vi "GUI Controller Performace Window.vi"() -> ()   [LabVIEW 2011, in "User Interface Window VIs.lvlib"]
uses:
  User Interface Window VIs.lvlib
  Types Definitions/Type Diagnostics Sample.ctl
  Types Definitions/Type Diagnostics Data.ctl
  Types Definitions/Type CPU Loads Array.ctl
  Types Definitions/Type CPU Loads.ctl
  Types Definitions/Type Configuration Data (GUI to Controller).ctl
  Types Definitions/Type FOFB Parameters.ctl
  Types Definitions/Type Network Configuration.ctl
  Types Definitions/Type FA Configuration.ctl
  Types Definitions/Type Response Matrix Measurement Configuration.ctl
  Types Definitions/Type Correction Algorithm Configuration.ctl
  Types Definitions/Type Acquisition Network Configuration.ctl
  Types Definitions/Type Actuation Network Configuration.ctl
  <vilib>/express/express shared/transition.llb/Dynamic To Waveform Array.vi
  <vilib>/express/express signal manip/GetorSetDDTAttributes/Set DDT Attributes/SetT0.vi
  <vilib>/express/express shared/transition.llb/Waveform Array To Dynamic.vi
  <vilib>/express/express signal manip/GetorSetDDTAttributes/Set DDT Attributes/Set DDT Properties.xnode
  Type Definitions.lvlib
panel:
  in  "Tab Control":T1(tab)
  out "Memory":dynamicdata(graph)=[{"t0"=timestamp(3442295670.8960543 s since 1904-01-01), "dt"=1.0, "Y"=[979.33984375], "attributes"=variant("NI_ExpTimeStamp"=variant(timestamp timestamp(3442295670.8960543 s since 1904-01-01)))}]
  out "Missed Iterations":dynamicdata(graph)=[{"t0"=timestamp(3442295670.8960543 s since 1904-01-01), "dt"=1.0, "Y"=[335.0], "attributes"=variant("NI_ExpTimeStamp"=variant(timestamp timestamp(3442295670.8960543 s since 1904-01-01)))}]
  out "CPU":dynamicdata(graph)=[{"t0"=timestamp(3442295670.8960543 s since 1904-01-01), "dt"=1.0, "Y"=[73.75901717969012], "attributes"=variant("NI_ExpTimeStamp"=variant(timestamp timestamp(3442295670.8960543 s since 1904-01-01)))}, {"t0"=timestamp(3442295670.8960543 s since 1904-01-01), "dt"=1.0, "Y"=[51.210817049644916], "attributes"=variant("NI_ExpTimeStamp"=variant(timestamp timestamp(3442295670.8960543 s since 1904-01-01)))}, {"t0"=timestamp(3442295670.8960543 s since 1904-01-01), "dt"=1.0, "Y"=[21.886355480263205], "attributes"=variant("NI_ExpTimeStamp"=variant(timestamp timestamp(3442295670.8960543 s since 1904-01-01)))}, {"t0"=timestamp(3442295670.8960543 s since 1904-01-01), "dt"=1.0, "Y"=[0.0], "attributes"=variant("NI_ExpTimeStamp"=variant(timestamp timestamp(3442295670.8960543 s since 1904-01-01)))}, {"t0"=timestamp(3442295670.8960543 s since 1904-01-01), "dt"=1.0, "Y"=[31.473643386938022], "attributes"=variant("NI_ExpTimeStamp"=variant(timestamp timestamp(3442295670.8960543 s since 1904-01-01)))}, {"t0"=timestamp(3442295670.8960543 s since 1904-01-01), "dt"=1.0, "Y"=[0.5343387174557266], "attributes"=variant("NI_ExpTimeStamp"=variant(timestamp timestamp(3442295670.8960543 s since 1904-01-01)))}, {"t0"=timestamp(3442295670.8960543 s since 1904-01-01), "dt"=1.0, "Y"=[30.632623496579622], "attributes"=variant("NI_ExpTimeStamp"=variant(timestamp timestamp(3442295670.8960543 s since 1904-01-01)))}, {"t0"=timestamp(3442295670.8960543 s since 1904-01-01), "dt"=1.0, "Y"=[0.0], "attributes"=variant("NI_ExpTimeStamp"=variant(timestamp timestamp(3442295670.8960543 s since 1904-01-01)))}]
  out "Execution Time":dynamicdata(graph)=[{"t0"=timestamp(3442295670.8960543 s since 1904-01-01), "dt"=1.0, "Y"=[0.0], "attributes"=variant("NI_ExpTimeStamp"=variant(timestamp timestamp(3442295670.8960543 s since 1904-01-01)))}]
  in  "Send RT Execution Trace Request":bool
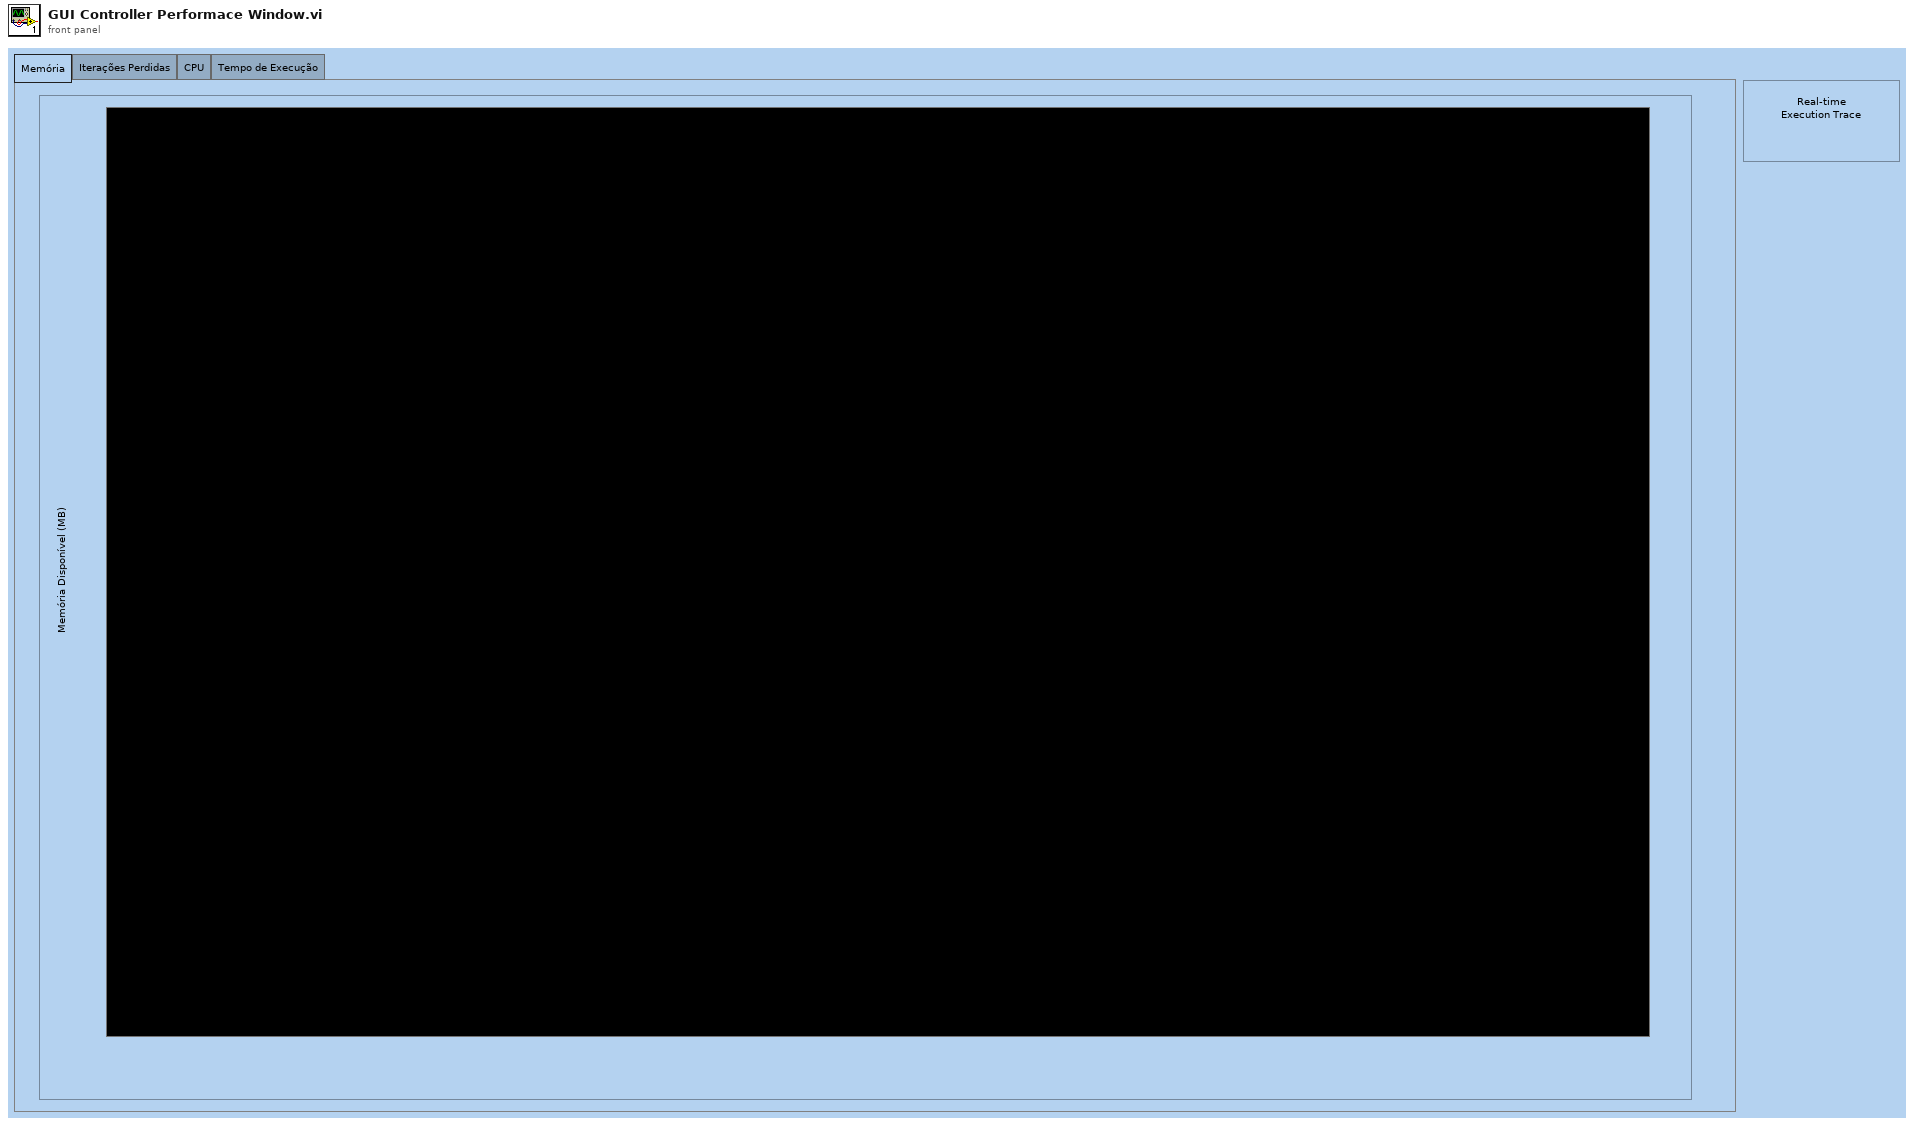
[diagram p1: front panel]
types:
  T1 = enum32{"Memória", "Iterações Perdidas", "CPU", "Tempo de Execução"}
  T2 = typedef "Type Definitions.lvlib/Type Configuration Data (GUI to Controller).ctl" = cluster{"Update Controller Soft Configuration":bool[], "Trigger RT Execution Trace":string[], "Reference Orbit":dbl[], "Request Response Matrix Folder List":bool[], "Request FOFB Parameters":bool[], "FOFB Parameters":T3[]}
  T3 = typedef "Type Definitions.lvlib/Type FOFB Parameters.ctl" = cluster{"Network":T4, "Fast Acquisition":T5, "Response Matrix Measurement":T6, "Correction Algorithm":T7, "Acquisition Network":T8, "Actuation Network":T9}
  T4 = typedef "Type Definitions.lvlib/Type Network Configuration.ctl" = cluster{"FOFB Controller IP":string, "LNLS Control Network IP":string, "LNLS Control Network Power Supplies TCP Port":u16, "LNLS Control Network FOFB Configuration TCP Port":u16, "Data Server TCP Port":u16, "Monitoring Data TCP Port":u16, "Configuration GUI TCP Port":u16, "TCP Listening Timeout":i32}
  T5 = typedef "Type Definitions.lvlib/Type FA Configuration.ctl" = cluster{"Acquisition Period":u32, "Data Buffer Size":u32, "Monitoring Period":u32}
  T6 = typedef "Type Definitions.lvlib/Type Response Matrix Measurement Configuration.ctl" = cluster{"Step Amplitude":dbl, "Time Between Steps":u32, "Step Duration":u32, "Number of Averages":u32}
  T7 = typedef "Type Definitions.lvlib/Type Correction Algorithm Configuration.ctl" = cluster{"Correction Period":u32, "Reference Orbit Path":path, "Response Matrix Path":path, "Correction Matrix Path":path, "Horizontal Correction Factor":dbl, "Vertical Correction Factor":dbl, "Beam Current FOFB Threshold":dbl, "Decouple H-V":bool, "Use Additional BPM LPF":bool, "BPM LPF Cutoff":dbl}
  T8 = typedef "Type Definitions.lvlib/Type Acquisition Network Configuration.ctl" = cluster{"Chassis Name":string, "Variables":cluster{"Variable Name":string, "Matrix Order":u32, "Location":dbl, "Plane":enum8{"H", "V"}, "On Correction":bool}[]}[]
  T9 = typedef "Type Definitions.lvlib/Type Actuation Network Configuration.ctl" = cluster{"Chassis Name":string, "Variables":cluster{"Variable Name":string, "Matrix Order":u32, "RMM Step Factor":dbl, "Plane":enum8{"H", "V"}, "On Correction":bool, "Kc":dbl, "Ti":dbl, "Td":dbl}[]}[]
  T10 = typedef "Type Definitions.lvlib/Type Diagnostics Sample.ctl" = cluster{"Timestamp":timestamp, "Diagnostics Data":T11}
  T11 = typedef "Type Definitions.lvlib/Type Diagnostics Data.ctl" = cluster{"Time-Critical Loop Missed Iterations":u32, "Time-Critical Loop Execution Time (usec)":u32, "FA Buffer Usage":u32, "Available Memory (bytes)":u32, "CPU Loads Array":T12}
  T12 = typedef "Type Definitions.lvlib/Type CPU Loads Array.ctl" = T13[]
  T13 = typedef "Type Definitions.lvlib/Type CPU Loads.ctl" = cluster{"Total (%)":dbl, "Time Critical (%)":dbl, "Timed Structures (%)":dbl, "High (%)":dbl, "Above Normal (%)":dbl, "Normal (%)":dbl, "Background (%)":dbl, "Idle (%)":dbl, "ISR (%)":dbl}
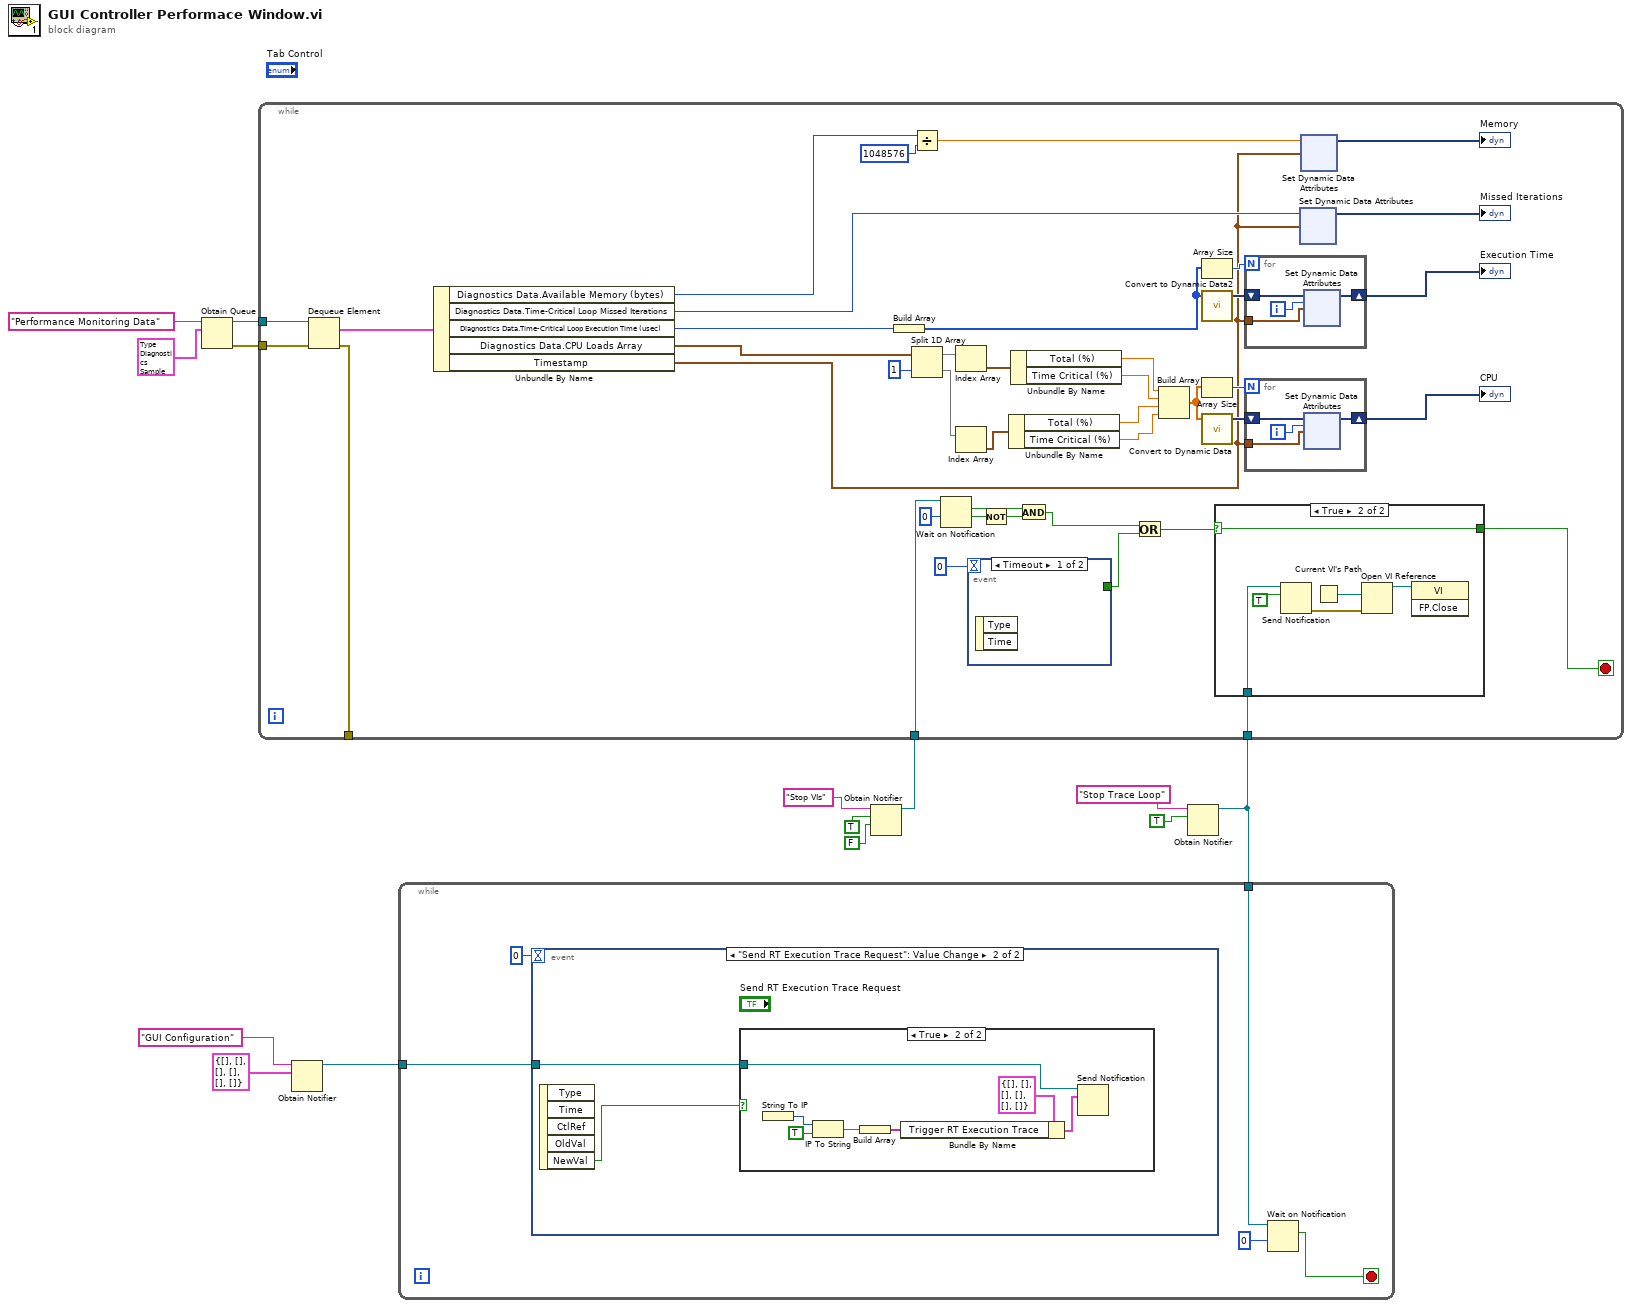
[diagram p0: block diagram]
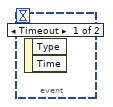
[diagram p2: hidden frame]
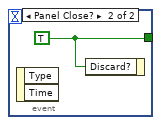
[diagram p5: hidden frame]
diagram:
  n1 = Obtain Queue(name (unnamed)="Performance Monitoring Data", element data type=T10 {"Timestamp"=timestamp(0 s since 1904-01-01), "Diagnostics Data"={"Time-Critical Loop Missed Iterations"=0, "Time-Critical Loop Execution Time (usec)"=0, "FA Buffer Usage"=0, "Available Memory (bytes)"=0, "CPU Loads Array"=[]}}) -> (queue out=w12:refnum<queue>, error out=w11:errorcluster)  [unwired: 3 in, 1 out]
  n2 = Obtain Notifier(name (unnamed)="GUI Configuration", notification data type=T2 {"Update Controller Soft Configuration"=[], "Trigger RT Execution Trace"=[], "Reference Orbit"=[], "Request Response Matrix Folder List"=[], "Request FOFB Parameters"=[], "FOFB Parameters"=[]} ("Configuration Data (GUI to Controller)")) -> (notifier out=w4:refnum<notifier>)  [unwired: 2 in, 2 out]
  n3 = Obtain Notifier(name (unnamed)="Stop VIs", notification data type=TRUE, create if not found? (T)=FALSE) -> (notifier out=w7:refnum<notifier>)  [unwired: 1 in, 2 out]
  n4 = Obtain Notifier(name (unnamed)="Stop Trace Loop", notification data type=TRUE ("notification")) -> (notifier out=w3:refnum<notifier>)  [unwired: 2 in, 2 out]
  n5 = while {
    tunnel: w12 -> [w39]
    tunnel: w11 -> [w38]
    tunnel: w7 -> [w28]
    tunnel: [w18] -> _
    tunnel: w3 -> [w17]
    stop <- w27 stop-if-true
    n6 = Dequeue Element(queue=w39, error in (no error)=w38) -> (element=w40:T10, error out=w18:errorcluster)  [unwired: 1 in, 2 out]
    n7 = Unbundle By Name(w40) -> ("Diagnostics Data.Available Memory (bytes)"=w21:u32, "Diagnostics Data.Time-Critical Loop Missed Iterations"=w25:u32, "Diagnostics Data.Time-Critical Loop Execution Time (usec)"=w37:u32, "Diagnostics Data.CPU Loads Array"=w24:T12, "Timestamp"=w22:timestamp)
    n8 = Build Array(w37) -> (w43:u32[])
    n9 = Divide(x=w21, y=u32 1048576) -> (x/y=w19:dbl)
    n10 = Split 1D Array(array=w24, index=1) -> (first subarray=w55:T12, second subarray=w53:T12)
    n11 = Wait on Notification(notifier=w28, timeout in ms (-1)=0) -> (notification=w32:bool, timed out?=w30:bool)  [unwired: 2 in, 2 out]
    n12 = Index Array(array=w55) -> (element=w54:T13)  [unwired: 1 in]
    n13 = Index Array(array=w53) -> (element=w52:T13)  [unwired: 1 in]
    n14 = event shown="[0] Timeout" {
      selector: _ -> [_ _]
      dyn-events: _ -> [_ _]
      timeout: 0 -> [_ _]
      tunnel: [_ w91] -> w35
      event Timeout {
        n15 = event-data() -> ()  [unwired: 1 in, 2 out]
      }
      event Panel Close? {
        w91 = TRUE
        n16 = event-data() -> ()  [unwired: 1 in, 2 out]
        n17 = event-data("Discard?"=w91) -> ()  [unwired: 1 in, 1 out]
      }
    }
    n18 = Not(x=w30) -> (.not. x?=w31:bool)
    n19 = Unbundle By Name(w52) -> ("Total (%)"=w16:dbl, "Time Critical (%)"=w15:dbl)
    n20 = Unbundle By Name(w54) -> ("Total (%)"=w51:dbl, "Time Critical (%)"=w50:dbl)
    n21 = And(x=w32, y=w31) -> (x .and. y?=w33:bool)
    n22 = Or(x=w33, y=w35) -> (x .or. y?=w36:bool)
    n23 = Build Array(w51, w50, w16, w15) -> (w45:dbl[])
    n24 = Array Size(array=w43) -> (size(s)=w44:i32)
    n25 = call "Convert to Dynamic Data2"("Array"=w43) -> ("Dynamic Data Type"=w42:dynamicdata)  [unwired: 3 in]
    n26 = Array Size(array=w45) -> (size(s)=w47:i32)
    n27 = call "Convert to Dynamic Data"("Array"=w45) -> ("Dynamic Data Type"=w48:dynamicdata)  [unwired: 3 in]
    n28 = case shown="True" w36 {
      selector: w36 -> [w84 w89]
      tunnel: [w84 w89] -> w27
      tunnel: w17 -> [_ w87]
      frame False {
      }
      frame True {
        n29 = Send Notification(notification=TRUE, notifier=w87) -> (error out=w85:errorcluster)  [unwired: 1 in, 1 out]
        n30 = Current VI's Path() -> (path=w88:path)
        n31 = Open VI Reference(vi path=w88, error in (no error)=w85) -> (vi reference=w90:refnum<vi>)  [unwired: 4 in, 1 out]
        n32 = invoke class="VI" method="FP.Close"(reference=w90) -> ()  [unwired: 2 in, 3 out]
      }
    }
    n33 = for {
      N: w44 -> [_]
      shift-right: [w95] -> w41
      shift-left: w42 -> [w93]
      tunnel: w22 -> [w92]
      i -> [w94]
      n34 = xnode ("Set Dynamic Data Attributes")("Signals In"=w93, "Signal Index"=w94, "Timestamp"=w92) -> ("Signals Out"=w95:dynamicdata)  [unwired: 1 in, 1 out]
    }
    "Execution Time" <- w41
    n35 = for {
      N: w47 -> [_]
      shift-right: [w112] -> w46
      shift-left: w48 -> [w110]
      tunnel: w22 -> [w109]
      i -> [w111]
      n36 = xnode ("Set Dynamic Data Attributes")("Signals In"=w110, "Signal Index"=w111, "Timestamp"=w109) -> ("Signals Out"=w112:dynamicdata)  [unwired: 1 in, 1 out]
    }
    "CPU" <- w46
    n37 = xnode ("Set Dynamic Data Attributes")("Signals In"=w25, "Timestamp"=w22) -> ("Signals Out"=→"Missed Iterations":dynamicdata)  [unwired: 2 in, 1 out]
    n38 = xnode ("Set Dynamic Data Attributes")("Signals In"=w19, "Timestamp"=w22) -> ("Signals Out"=→"Memory":dynamicdata)  [unwired: 2 in, 1 out]
  }
  n39 = while {
    tunnel: w4 -> [w130]
    tunnel: w3 -> [w129]
    stop <- w128 stop-if-true
    n40 = event shown="[1] \"Send RT Execution Trace Request\": Value Change" {
      selector: _ -> [_ _]
      dyn-events: _ -> [_ _]
      timeout: 0 -> [_ _]
      tunnel: w130 -> [_ w132]
      event Timeout {
        n41 = event-data() -> ()  [unwired: 1 in, 2 out]
      }
      event "Send RT Execution Trace Request": Value Change {
        n42 = event-data() -> ("NewVal"=w131:bool)  [unwired: 1 in, 4 out]
        n43 = case shown="True" w131 {
          tunnel: w132 -> [_ w133]
          frame False {
          }
          frame True {
            n44 = String To IP() -> (0:w138:u32)  [unwired: 1 in]
            n45 = IP To String(1:TRUE ("dot notation? (F)"), 2:w138) -> (0:w136:string)
            n46 = Build Array(w136) -> (w139:string[])
            n47 = Bundle By Name(cluster=T2 {"Update Controller Soft Configuration"=[], "Trigger RT Execution Trace"=[], "Reference Orbit"=[], "Request Response Matrix Folder List"=[], "Request FOFB Parameters"=[], "FOFB Parameters"=[]} ("notification"), "Trigger RT Execution Trace"=w139) -> (w134:T2)
            n48 = Send Notification(notification=w134, notifier=w133) -> ()  [unwired: 1 in, 2 out]
          }
        }
      }
    }
    n49 = Wait on Notification(notifier=w129, timeout in ms (-1)=0) -> (notification=w128:bool)  [unwired: 2 in, 3 out]
  }
